vi "Pressure Conversion.vi"(10 "Waveform in":waveform(dbl)) -> (1 "Status":string, 2 "Waveform out":waveform(dbl))   [LabVIEW 2021, in "BPG.lvclass"]
uses:
  BPG.lvclass
  BPG.lvclass/BPG.ctl
  <vilib>/Analysis/NI_AALBase.lvlib
  <vilib>/Analysis/baseanly.llb/Mean (DBL).vi
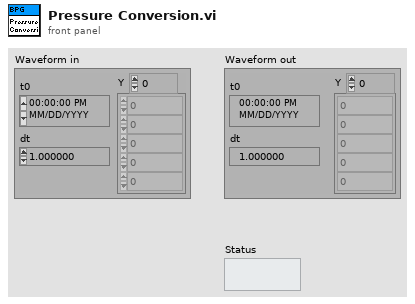
[diagram p1: front panel]
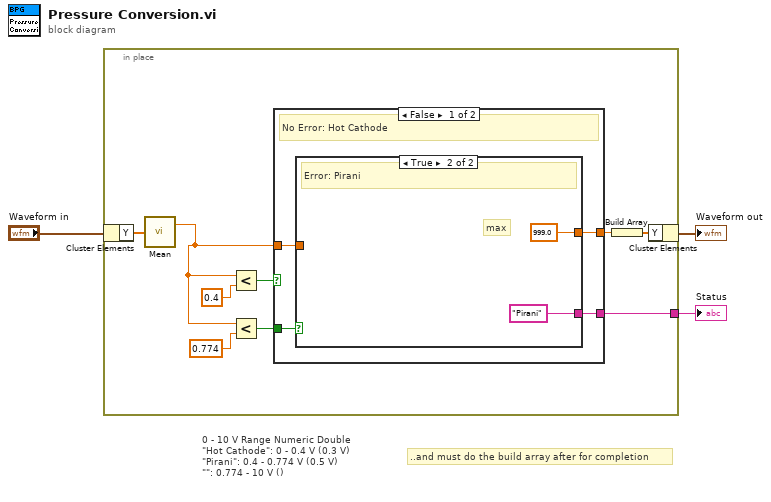
[diagram p0: block diagram]
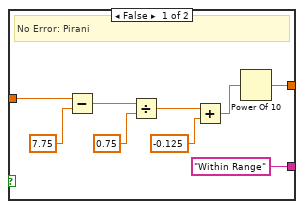
[diagram p2: hidden frame]
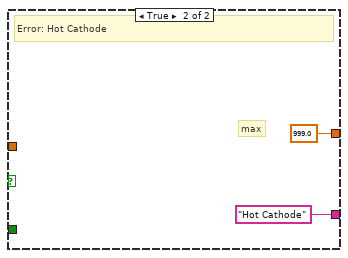
[diagram p3: hidden frame]
diagram:
  # "..and must do the build array after for completion"
  # "0 - 10 V Range Numeric Double\n\"Hot Cathode\": 0 - 0.4 V (0.3 V)\n\"Pirani\": 0.4 - 0.774 V (0.5 V)\n\"\": 0.774 - 10 V ()"
  n1 = in-place {
    in-place-border: [w12] -> w1
    n2 = in-place-cluster #1("Waveform in") -> ("Y"=w5:dbl[])
    n3 = call-poly <vilib>:"Mean.vi"("X"=w5) -> ("mean"=w4:dbl)  [unwired: 1 out]
    n4 = Less?(x=w4, y=0.4) -> (x < y?=w9:bool)
    n5 = Less?(x=w4, y=0.774) -> (x < y?=w10:bool)
    n6 = case shown="False" w9 {
      tunnel: w10 -> [w16 _]
      tunnel: [w15 999.0] -> w11
      tunnel: w4 -> [w14 _]
      tunnel: [w13 "Hot Cathode"] -> w12
      frame False {
        # "No Error: Hot Cathode"
        n7 = case shown="True" w16 {
          tunnel: [w25 999.0] -> w15
          tunnel: w14 -> [w24 _]
          tunnel: ["Within Range" "Pirani"] -> w13
          frame False {
            # "No Error: Pirani"
            n8 = Subtract(x=w24, y=7.75) -> (x-y=w22:dbl)
            n9 = Divide(x=w22, y=0.75) -> (x/y=w20:dbl)
            n10 = Add(x=w20, y=-0.125) -> (x+y=w18:dbl)
            n11 = Power Of 10(x=w18) -> (10^x=w25:dbl)
          }
          frame True {
            # "max"
            # "Error: Pirani"
          }
        }
      }
      frame True {
        # "max"
        # "Error: Hot Cathode"
      }
    }
    n12 = Build Array(w11) -> (w6:dbl[])
    n13 = in-place-cluster #1("Y"=w6) -> (→"Waveform out":waveform(dbl))
  }
  "Status" <- w1
